vi "Queue Driver.vi"(0 "States":string[](array[string]), 11 "Error In":errorcluster, 13 "Queue Operation":T1) -> (4 "Dequeue Element":string, 15 "Error Out":errorcluster)   [LabVIEW 2020, in "DNL INL Test.lvlib"]
doc: "Queue driver to store and execute the set of states."
uses:
  DNL INL Test.lvlib
  Typedef/Queue Operation.ctl
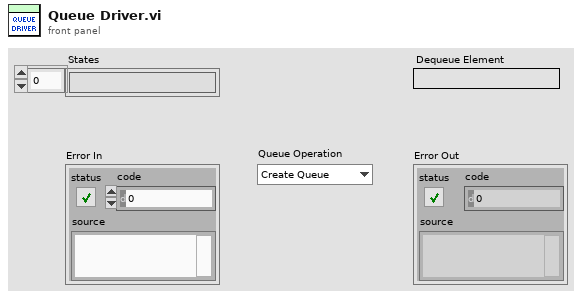
[diagram p1: front panel]
types:
  T1 = typedef "DNL INL Test.lvlib/Queue Operation.ctl" = enum16{"Create Queue", "Enqueue", "Dequeue", "Enstack", "Flush Queue", "Release Queue"}
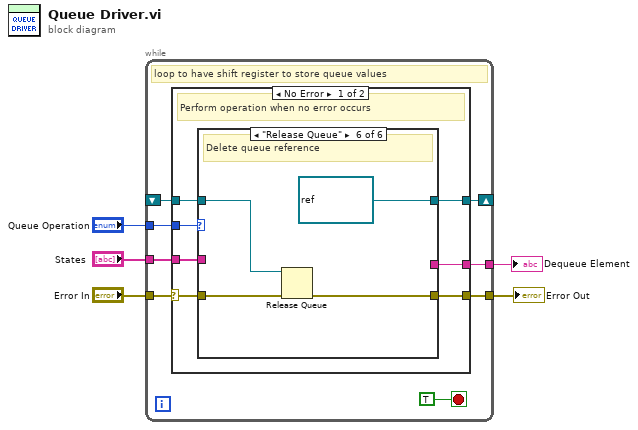
[diagram p0: block diagram]
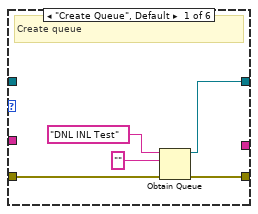
[diagram p2: hidden frame]
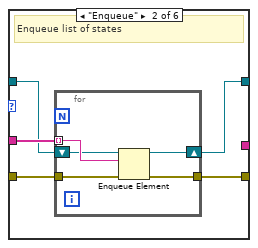
[diagram p3: hidden frame]
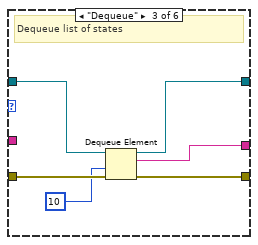
[diagram p4: hidden frame]
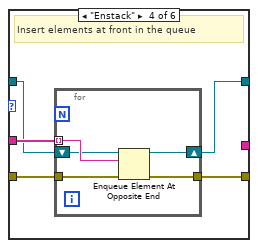
[diagram p5: hidden frame]
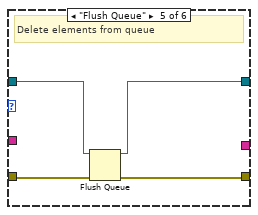
[diagram p6: hidden frame]
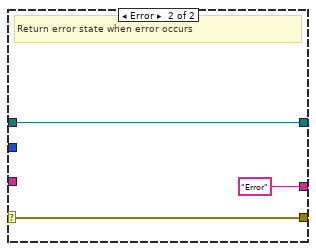
[diagram p7: hidden frame]
diagram:
  n1 = while {
    tunnel: "Error In" -> [w13]
    tunnel: "Queue Operation" -> [w12]
    tunnel: [w11] -> w3
    shift-right: [w10] -> _
    shift-left: _ -> [w8]
    tunnel: "States" -> [w9]
    tunnel: [w7] -> w1
    stop <- TRUE stop-if-true
    # "loop to have shift register to store queue values"
    n2 = case shown="No Error" w13 {
      selector: w13 -> [w19 w60]
      tunnel: w12 -> [w20 _]
      tunnel: [w18 w60] -> w11
      tunnel: [w17 w62] -> w10
      tunnel: w9 -> [w16 _]
      tunnel: w8 -> [w15 w62]
      tunnel: [w14 "Error"] -> w7
      frame No Error {
        # "Perform operation when no error occurs"
        n3 = case shown="\"Release Queue\"" w20 {
          tunnel: w19 -> [w25 w30 w41 w46 w55 w59]
          tunnel: [w22 w27 w39 w43 w54 w56] -> w18
          tunnel: [w21 w26 w38 w42 w53 refnum<queue> refnum ("queue out")] -> w17
          tunnel: w16 -> [_ w29 _ w45 _ _]
          tunnel: w15 -> [_ w28 w40 w44 w52 w58]
          tunnel: [_ _ w37 _ _ _] -> w14
          frame "Create Queue", Default {
            # "Create queue"
            n4 = Obtain Queue(name (unnamed)="DNL INL Test", element data type="", error in (no error)=w25) -> (queue out=w21:refnum<queue>, error out=w22:errorcluster)  [unwired: 2 in, 1 out]
          }
          frame "Enqueue" {
            # "Enqueue list of states"
            n5 = for {
              tunnel: w30 -> [w35]
              tunnel: w29 -> [w34] mode=indexing
              tunnel: [w32] -> w27
              shift-right: [w31] -> w26
              shift-left: w28 -> [w33]
              n6 = Enqueue Element(queue=w33, element=w34, error in (no error)=w35) -> (queue out=w31:refnum<queue>, error out=w32:errorcluster)  [unwired: 1 in, 1 out]
            }
          }
          frame "Dequeue" {
            # "Dequeue list of states"
            n7 = Dequeue Element(queue=w40, timeout in ms (-1)=10, error in (no error)=w41) -> (queue out=w38:refnum<queue>, element=w37:string, error out=w39:errorcluster)  [unwired: 1 out]
          }
          frame "Enstack" {
            # "Insert elements at front in the queue"
            n8 = for {
              tunnel: w46 -> [w51]
              tunnel: w45 -> [w50] mode=indexing
              tunnel: [w48] -> w43
              shift-right: [w47] -> w42
              shift-left: w44 -> [w49]
              n9 = Enqueue Element At Opposite End(queue=w49, element=w50, error in (no error)=w51) -> (queue out=w47:refnum<queue>, error out=w48:errorcluster)  [unwired: 1 in, 1 out]
            }
          }
          frame "Flush Queue" {
            # "Delete elements from queue"
            n10 = Flush Queue(queue=w52, error in (no error)=w55) -> (queue out=w53:refnum<queue>, error out=w54:errorcluster)  [unwired: 1 out]
          }
          frame "Release Queue" {
            # "Delete queue reference"
            n11 = Release Queue(queue=w58, error in (no error)=w59) -> (error out=w56:errorcluster)  [unwired: 1 in, 2 out]
          }
        }
      }
      frame Error {
        # "Return error state when error occurs"
      }
    }
  }
  "Error Out" <- w3
  "Dequeue Element" <- w1
